vi "rvc 2D Euler to Homogeneous (scalar).vi"(8 "error in (no error)":errorcluster, 10 "y":dbl, 11 "x":dbl) -> (0 "Error Out":errorcluster, 3 "Homogeneous":T1)   [LabVIEW 2013]
uses:
  <vilib>/Analysis/Matrix/Datatypes/RealMatrix.ctl
  <vilib>/Analysis/Matrix/NI_Matrix.lvlib
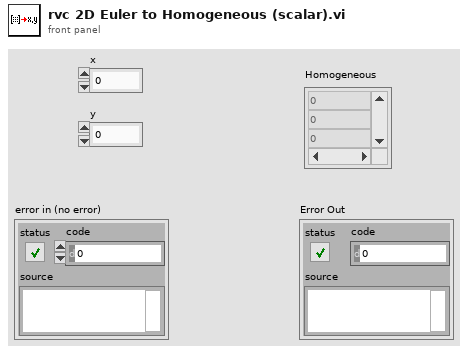
[diagram p1: front panel]
types:
  T1 = typedef "NI_Matrix.lvlib/RealMatrix.ctl" = dbl[][]
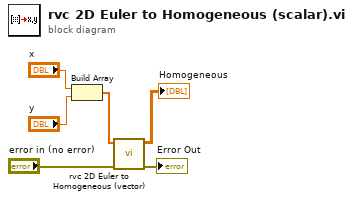
[diagram p0: block diagram]
diagram:
  n1 = Build Array("x", "y") -> (w4:dbl[])
  n2 = call "rvc 2D Euler to Homogeneous (vector).vi"("error in (no error)"="error in (no error)", "Euler"=w4) -> ("Error Out"=→"Error Out":errorcluster, "Homogeneous"=→"Homogeneous":T1)  [unwired: 8 in]
